vi "stimulus panel.vi"() -> (2 "stimulus setup":T1)   [LabVIEW 2018]
uses:
  global.vi
panel:
  in  "保存":T2
  in  "更新信号":T2
  in  "信号幅值(V)":dbl
  in  "频率上限(Hz)":dbl
  in  "频率下限(Hz)":dbl
  in  "信号时长(s)":dbl
  out "Waveform":waveform(dbl)(graph)
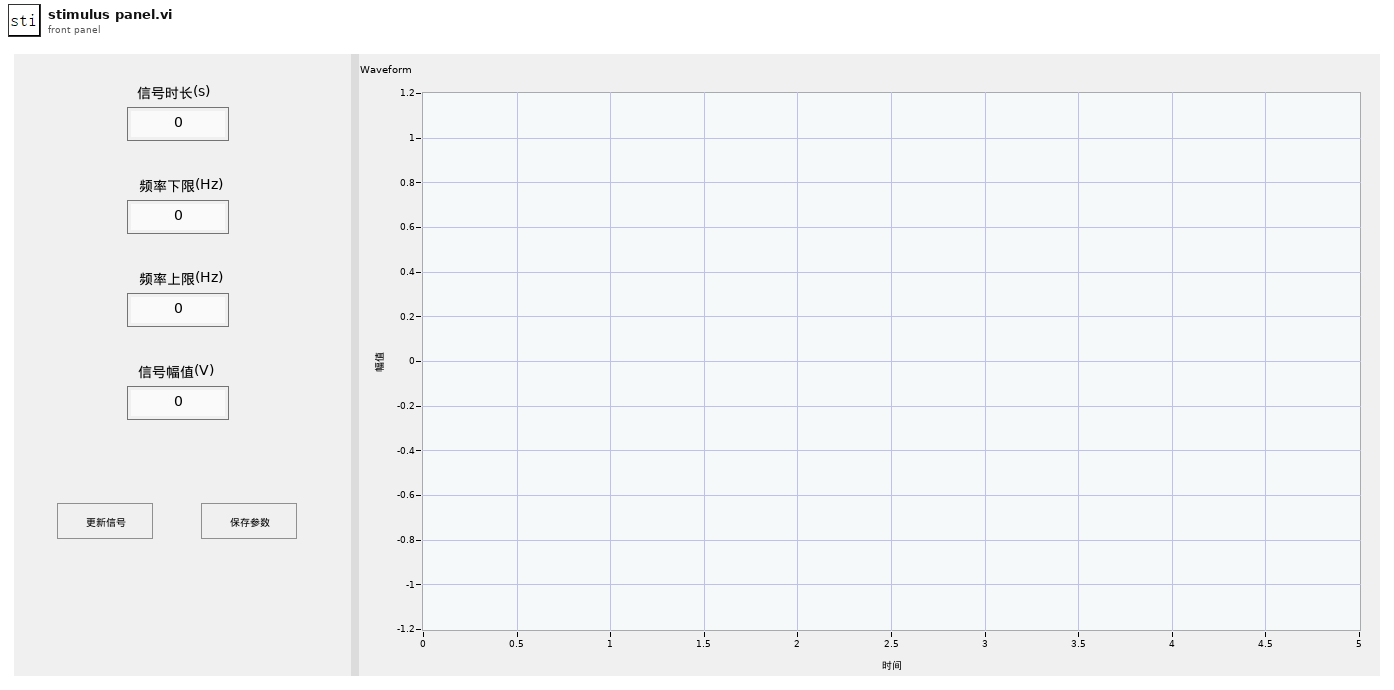
[diagram p1: front panel]
types:
  T1 = cluster{"幅值(V)":dbl, "信号时长(s)":dbl, "频率上限(Hz)":dbl, "频率下限(Hz)":dbl}
  T2 = typedef "布尔控件.ctl" = bool
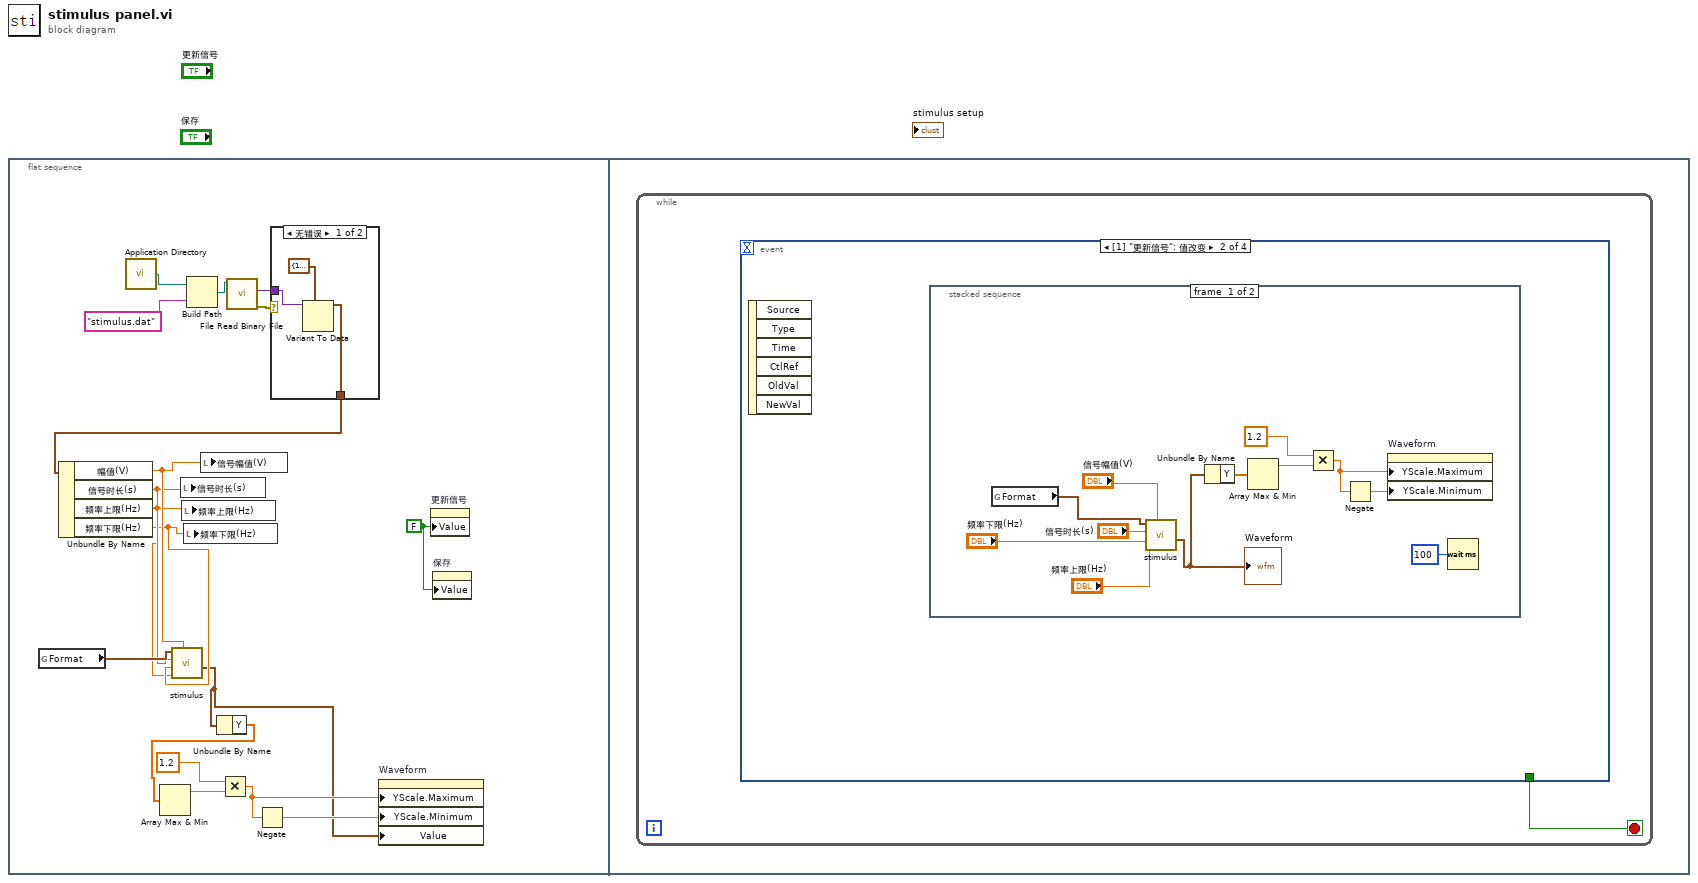
[diagram p0: block diagram]
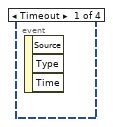
[diagram p3: hidden frame]
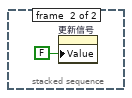
[diagram p4: hidden frame]
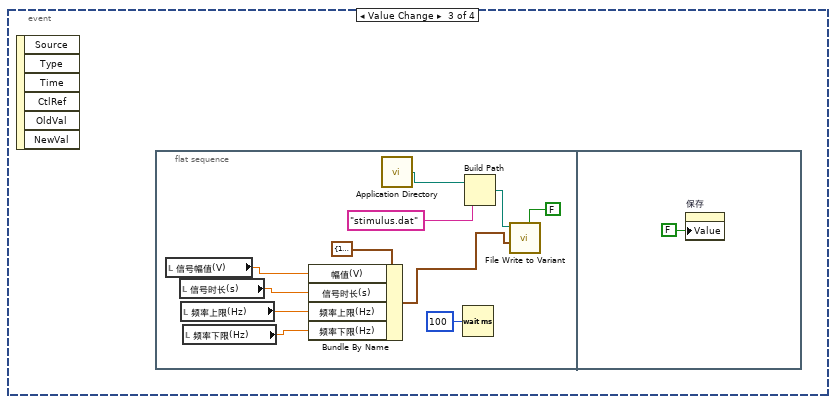
[diagram p5: hidden frame]
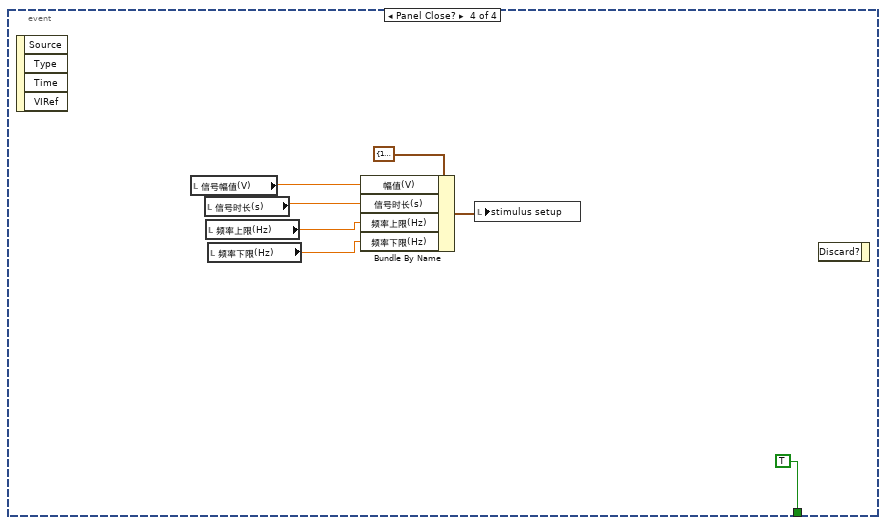
[diagram p6: hidden frame]
diagram:
  n1 = flat-sequence {
    frame #0 {
      w18 = T2 FALSE ("更新信号")
      n2 = global read "global.vi" "Format"() -> (w10:cluster{"Rate":i32, "Bits":i32, "Channels":u32})
      n3 = call <vilib>:"Application Directory.vi"() -> ("Application Directory"=w12:path)
      n4 = Build Path(base path=w12, name or relative path="stimulus.dat" ("名称或相对路径")) -> (appended path=w16:path)
      n5 = call "File Read Binary File.vi"("file path"=w16) -> ("error Output"=w15:errorcluster, "Variant Output"=w14:variant)  [unwired: 8 in, 1 out]
      n6 = case shown="无错误" w15 {
        tunnel: w14 -> [w21 _]
        tunnel: [w19 _] -> w13
        frame No Error {
          n7 = Variant To Data(type=T1 {"幅值(V)"=1.0, "信号时长(s)"=3.0, "频率上限(Hz)"=20000.0, "频率下限(Hz)"=10.0} ("stimulus setup"), Variant=w21) -> (data=w19:T1)  [unwired: 1 in, 1 out]
        }
        frame Error {
        }
      }
      n8 = Unbundle By Name(w13) -> ("幅值(V)"=w11:dbl, "信号时长(s)"=w9:dbl, "频率上限(Hz)"=w7:dbl, "频率下限(Hz)"=w8:dbl)
      n9 = call "stimulus.vi"("幅值(V)"=w11, "stop frequency [Hz]"=w7, "start frequency [Hz]"=w8, "信号时长"=w9, "Format"=w10) -> ("stimulus"=w1:waveform(dbl))  [unwired: 3 in, 3 out]
      n10 = local write "信号时长(s)"(w9) -> ()
      n11 = local write "频率上限(Hz)"(w7) -> ()
      n12 = local write "频率下限(Hz)"(w8) -> ()
      n13 = local write "信号幅值(V)"(w11) -> ()
      n14 = Unbundle By Name(w1) -> ("Y"=w2:dbl[])
      n15 = Array Max & Min(array=w2) -> (max value=w3:dbl)  [unwired: 3 out]
      n16 = Multiply(x=1.2, y=w3) -> (x*y=w5:dbl)
      n17 = Negate(x=w5) -> (-x=w6:dbl)
      n18 = property on="Waveform" class="WFGraph (严格)"("YScale.Maximum"=w5, "YScale.Minimum"=w6, "Value"=w1) -> ()  [unwired: 2 in, 2 out]
      n19 = property on="更新信号" class="Bool (严格)"("Value"=w18) -> ()  [unwired: 2 in, 2 out]
      n20 = property on="保存" class="Bool (严格)"("Value"=w18) -> ()  [unwired: 2 in, 2 out]
    }
    frame #1 {
      n21 = while {
        stop <- w22 stop-if-true
        n22 = event shown="[1] \"更新信号\": 值改变" {
          selector: _ -> [_ _ _ _]
          dyn-events: _ -> [_ _ _ _]
          timeout: _ -> [_ _ _ _]
          tunnel: [_ _ _ TRUE] -> w22
          event Timeout {
            n23 = event-data() -> ()  [unwired: 1 in, 3 out]
          }
          event Value Change {
            n24 = event-data() -> ()  [unwired: 1 in, 6 out]
            n25 = stacked-sequence {
              frame #0 {
                n26 = global read "global.vi" "Format"() -> (w34:cluster{"Rate":i32, "Bits":i32, "Channels":u32})
                n27 = call "stimulus.vi"("幅值(V)"="信号幅值(V)", "stop frequency [Hz]"="频率上限(Hz)", "start frequency [Hz]"="频率下限(Hz)", "信号时长"="信号时长(s)", "Format"=w34) -> ("stimulus"=w28:waveform(dbl))  [unwired: 3 in, 3 out]
                "Waveform" <- w28
                n28 = Unbundle By Name(w28) -> ("Y"=w27:dbl[])
                n29 = Array Max & Min(array=w27) -> (max value=w26:dbl)  [unwired: 3 out]
                n30 = Multiply(x=1.2, y=w26) -> (x*y=w24:dbl)
                n31 = Negate(x=w24) -> (-x=w23:dbl)
                n32 = property on="Waveform" class="WFGraph (严格)"("YScale.Maximum"=w24, "YScale.Minimum"=w23) -> ()  [unwired: 2 in, 2 out]
                n33 = Wait (ms)(milliseconds to wait=u32 100 ("等待时间（毫秒）")) -> ()  [unwired: 1 out]
              }
              frame #1 {
                n34 = property on="更新信号" class="Bool (严格)"("Value"=T2 FALSE ("更新信号")) -> ()  [unwired: 2 in, 2 out]
              }
            }
          }
          event Value Change {
            n35 = event-data() -> ()  [unwired: 1 in, 6 out]
            n36 = flat-sequence {
              frame #0 {
                n37 = local read "信号幅值(V)"() -> (w39:dbl)
                n38 = local read "信号时长(s)"() -> (w38:dbl)
                n39 = local read "频率上限(Hz)"() -> (w37:dbl)
                n40 = local read "频率下限(Hz)"() -> (w36:dbl)
                n41 = Bundle By Name(cluster=T1 {"幅值(V)"=1.0, "信号时长(s)"=3.0, "频率上限(Hz)"=20000.0, "频率下限(Hz)"=20.0} ("输入簇"), "幅值(V)"=w39, "信号时长(s)"=w38, "频率上限(Hz)"=w37, "频率下限(Hz)"=w36) -> (w40:T1)
                n42 = call <vilib>:"Application Directory.vi"() -> ("Application Directory"=w42:path)
                n43 = Wait (ms)(milliseconds to wait=u32 100 ("等待时间（毫秒）")) -> ()  [unwired: 1 out]
                n44 = Build Path(base path=w42, name or relative path="stimulus.dat" ("名称或相对路径")) -> (appended path=w45:path)
                n45 = call "File Write to Variant.vi"("替换提示"=FALSE, "Input Data"=w40, "Path to Write"=w45) -> ()  [unwired: 4 in, 5 out]
              }
              frame #1 {
                n46 = property on="保存" class="Bool (严格)"("Value"=T2 FALSE ("保存")) -> ()  [unwired: 2 in, 2 out]
              }
            }
          }
          event Panel Close? {
            n47 = event-data() -> ()  [unwired: 1 in, 4 out]
            n48 = local read "信号幅值(V)"() -> (w52:dbl)
            n49 = local read "信号时长(s)"() -> (w51:dbl)
            n50 = local read "频率上限(Hz)"() -> (w50:dbl)
            n51 = local read "频率下限(Hz)"() -> (w49:dbl)
            n52 = Bundle By Name(cluster=T1 {"幅值(V)"=1.0, "信号时长(s)"=3.0, "频率上限(Hz)"=20000.0, "频率下限(Hz)"=10.0} ("stimulus setup"), "幅值(V)"=w52, "信号时长(s)"=w51, "频率上限(Hz)"=w50, "频率下限(Hz)"=w49) -> (w48:T1)
            n53 = local write "stimulus setup"(w48) -> ()
            n54 = event-data() -> ()  [unwired: 2 in, 1 out]
          }
        }
      }
    }
  }
